vi "EnumInterfaces.vi"(8 "error in (no error)":errorcluster, 9 "nTLayerType":u32) -> (0 "error out":errorcluster, 1 "pInterfaceInfoList":T1(array[cluster]), 2 "return type":i32 format="%x")   [LabVIEW 2013, in "MvCameraControl.lvlib"]
doc: "MV_CAMCTRL_API int __stdcall MV_CC_EnumInterfaces(IN unsigned int nTLayerType, IN OUT MV_INTERFACE_INFO_LIST* pInterfaceInfoList);"
uses:
  MvCameraControl.lvlib
  MvCameraPatch.dll
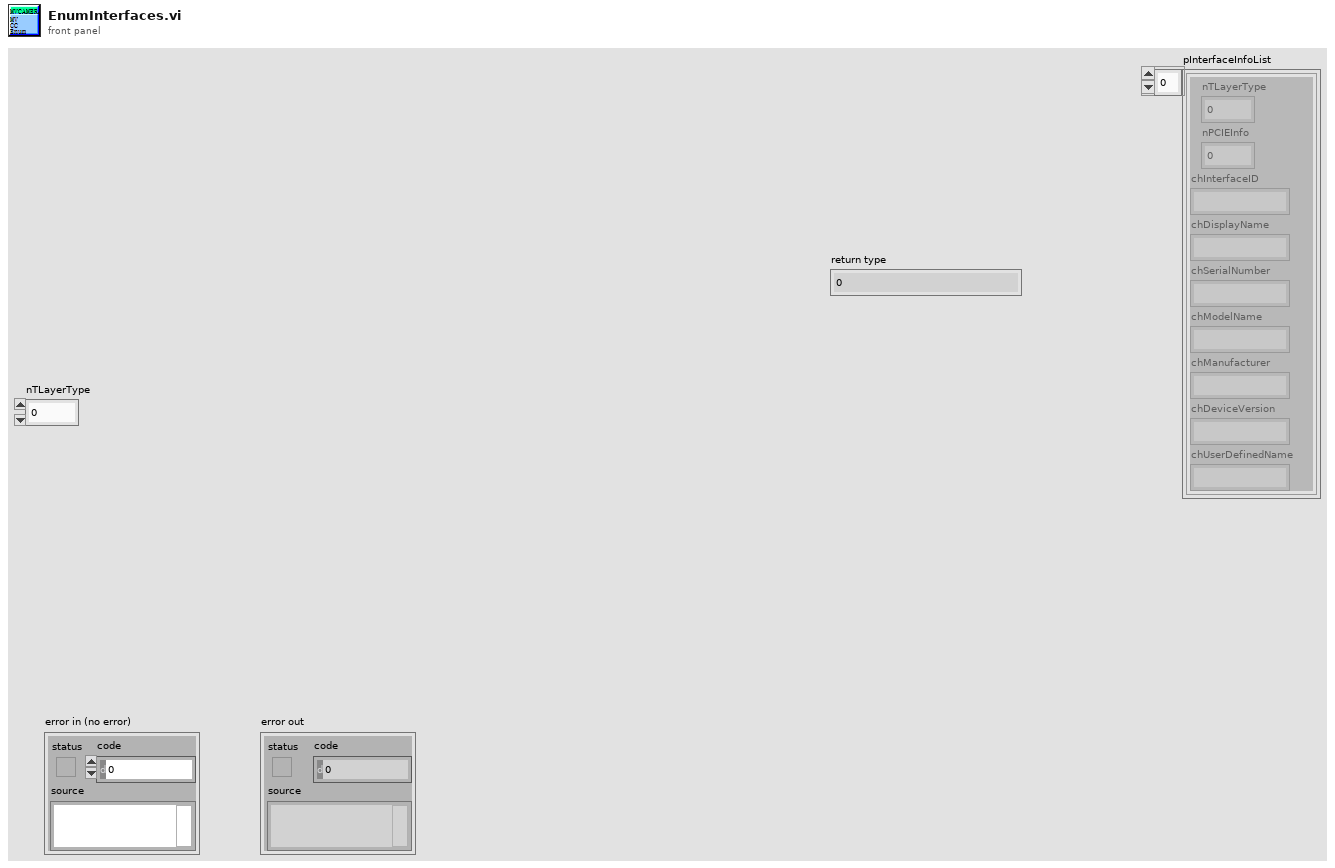
[diagram p1: front panel]
types:
  T1 = cluster{"nTLayerType":u32, "nPCIEInfo":u32, "chInterfaceID":string, "chDisplayName":string, "chSerialNumber":string, "chModelName":string, "chManufacturer":string, "chDeviceVersion":string, "chUserDefinedName":string}[]
  T2 = cluster{"nTLayerType":u32, "nPCIEInfo":u32, "chInterfaceID":string, "chDisplayName":string, "chSerialNumber":string, "chModelName":string, "chManufacturer":string, "chDeviceVersion":string, "chUserDefinedName":string}
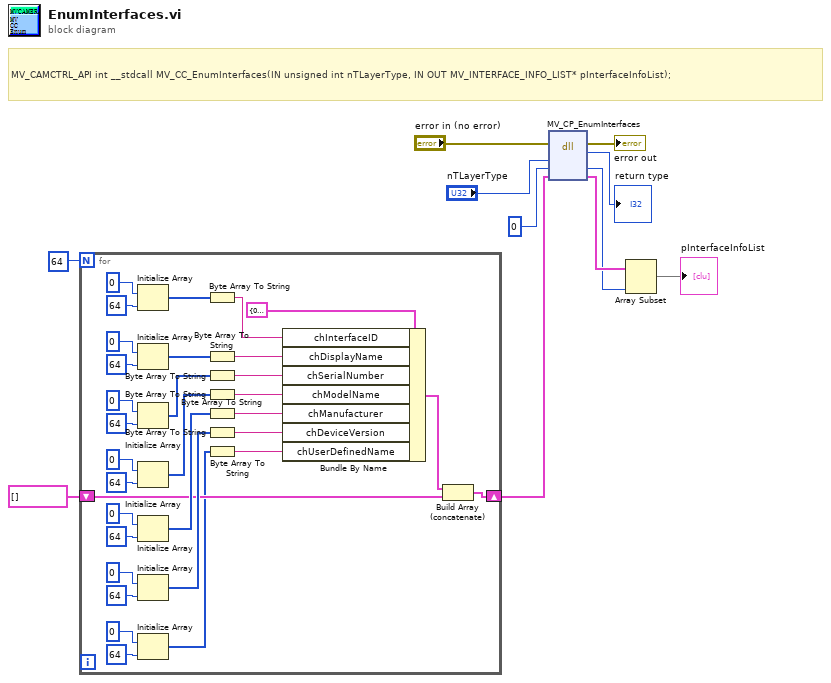
[diagram p0: block diagram]
diagram:
  # "MV_CAMCTRL_API int __stdcall MV_CC_EnumInterfaces(IN unsigned int nTLayerType, IN OUT MV_INTERFACE_INFO_LIST* pInterfaceInfoList);"
  n1 = for {
    N: 64 -> [_]
    shift-right: [w21] -> w4
    shift-left: T1 [] -> [w19]
    n2 = Initialize Array(u8 0 ("元素"), 64 ("维数大小")) -> (w29:u8[])
    n3 = Initialize Array(u8 0 ("元素"), 64 ("维数大小")) -> (w32:u8[])
    n4 = Initialize Array(u8 0 ("元素"), 64 ("维数大小")) -> (w22:u8[])
    n5 = Initialize Array(u8 0 ("元素"), 64 ("维数大小")) -> (w26:u8[])
    n6 = Initialize Array(u8 0 ("元素"), 64 ("维数大小")) -> (w40:u8[])
    n7 = Initialize Array(u8 0 ("元素"), 64 ("维数大小")) -> (w37:u8[])
    n8 = Initialize Array(u8 0 ("元素"), 64 ("维数大小")) -> (w13:u8[])
    n9 = Byte Array To String(unsigned byte array=w29) -> (string=w17:string)
    n10 = Byte Array To String(unsigned byte array=w32) -> (string=w41:string)
    n11 = Byte Array To String(unsigned byte array=w22) -> (string=w23:string)
    n12 = Byte Array To String(unsigned byte array=w26) -> (string=w16:string)
    n13 = Byte Array To String(unsigned byte array=w40) -> (string=w42:string)
    n14 = Byte Array To String(unsigned byte array=w37) -> (string=w43:string)
    n15 = Byte Array To String(unsigned byte array=w13) -> (string=w12:string)
    n16 = Bundle By Name(cluster=T2 {"nTLayerType"=0, "nPCIEInfo"=0, "chInterfaceID"="", "chDisplayName"="", "chSerialNumber"="", "chModelName"="", "chManufacturer"="", "chDeviceVersion"="", "chUserDefinedName"=""} ("InterfaceInfo"), "chInterfaceID"=w17, "chDisplayName"=w41, "chSerialNumber"=w23, "chModelName"=w16, "chManufacturer"=w42, "chDeviceVersion"=w43, "chUserDefinedName"=w12) -> (w20:T2)
    n17 = Build Array (concatenate)(w20, w19) -> (w21:T1)
  }
  n18 = dll-call lib="MvCameraPatch.dll" fn="MV_CP_EnumInterfaces"(error in="error in (no error)", "nTLayerType"="nTLayerType", "nInterfaceNum"=u32 0, "pInterfaceInfoList"=w4) -> (error out=→"error out":errorcluster, "return type"=→"return type":i32, "nInterfaceNum"=w2:u32, "pInterfaceInfoList"=w3:T1)  [unwired: 3 in, 1 out]
  n19 = Array Subset(array=w3, length=w2) -> (→"pInterfaceInfoList":T1)  [unwired: 1 in]
